vi "Host_FastOsziTest_backup.vi"() -> ()   [LabVIEW 2012]
uses:
  <vilib>/FPGAPlugInAG/PXIe-7962R/niLvFpga_Open_PXIe-7962R.vi
  <vilib>/rvi/interface/common/dynamic/niFpgaDynamicAddResources.vi
  <vilib>/Utility/error.llb/Error Cluster From Error Code.vi
  <vilib>/rvi/errors/niLvFpgaAdjustHostInterfaceError.vi
  <vilib>/FPGAPlugInAG/Dynamic/niLvFpga_Close_Dynamic.vi
  <vilib>/rvi/interface/nirviOpenFPGA/nirviOpenFPGA.xnode
  FPGA Bitfiles/AnalogIntegratorFastOszi_NI5771_PXIe-7962R.lvbitx
  <vilib>/rvi/interface/nirviReadWriteControl/nirviReadWriteControl.xnode
  <vilib>/rvi/interface/nirviMethod/nirviMethod.xnode
  <vilib>/rvi/interface/nirviCloseFPGA/nirviCloseFPGA.xnode
  <vilib>/rvi/interface/Simulation/niFpgaSimulationCallBeginRW.vi
  NiFpgaLv.dll
  <vilib>/FPGAPlugInAG/Dynamic/niLvFpga_ReadFifo_Dynamic.vi
  <vilib>/rvi/errors/niLvFpgaMergeErrorWithErrorCode.vi
  <vilib>/Analysis/NI_AALPro.lvlib
panel:
  in  "Baseline Subtract":u8=16
  in  "Pixels to Integrate":u32=10000
  in  "stop 3":bool
  out "NOT Crosstalk":dbl format="%0.2f"
  out "Crosstalk":dbl format="%0.2f"
  in  "Save?":bool
  out "time to draw(ms) 2":i32=1000
  out "Area 1":picture
  in  "stop 2":bool
  in  "sized scatter plot cosmetics 2":T1={"min size"=1, "max size"=5, "maps to max size"=5, "color array"=[16711680, 65280, 255, 16776960, 16737792, 65535]}
  in  "cartesian axis attributes 2":T2={"x minimum"=1.0, "x maximum"=500.0, "x log?"=FALSE, "x precision"=1, "x format"=enum."Decimal", "y minimum"=60.0, "y maximum"=740.0, "y log?"=FALSE, "y precision"=1, "y format"=enum."Decimal"} {"x minimum" format="%0.2f"; "x maximum" format="%0.2f"; "y minimum" format="%0.2f"; "y maximum" format="%0.2f"}
  in  "?":u16(ring)=4 items=["Points", "Squares", "Circles", "Sized Squares", "Sized-Colored Squares", "Min-Max Lines"]
  in  "line color 2":u32(colorbox)=39168
  in  "text color 2":u32(colorbox)=65280
  in  "plot color 2":u32(colorbox)=16776960
  out "time to draw(ms)":i32=1000
  out "Area 2":picture
  in  "stop":bool
  in  "sized scatter plot cosmetics":T1={"min size"=1, "max size"=5, "maps to max size"=5, "color array"=[16711680, 65280, 255, 16776960, 16737792, 65535]}
  in  "cartesian axis attributes":T2={"x minimum"=1.0, "x maximum"=500.0, "x log?"=FALSE, "x precision"=1, "x format"=enum."Decimal", "y minimum"=60.0, "y maximum"=740.0, "y log?"=FALSE, "y precision"=1, "y format"=enum."Decimal"} {"x minimum" format="%0.2f"; "x maximum" format="%0.2f"; "y minimum" format="%0.2f"; "y maximum" format="%0.2f"}
  in  "?":u16(ring)=4 items=["Points", "Squares", "Circles", "Sized Squares", "Sized-Colored Squares", "Min-Max Lines"]
  in  "line color":u32(colorbox)=39168
  in  "text color":u32(colorbox)=65280
  in  "plot color":u32(colorbox)=16776960
  out "PMT histogram":T3(graph)
  out "Mean NOT pulse length":dbl format="%0.2f"
  out "Mean pulse length":dbl format="%0.2f"
  out "NOT Laser pulse length histogram":T3(graph)
  out "Laser pulse length histogram":T3(graph)
  out "Laser (Trigger In)":i16[](graph)
  in  "Samples per Pixels":u32=10000
  out "IO Module\\AI Over Range":bool
  out "PMT (AI 0)":u8[](graph)
  # "Sampling at 1.5GHz => 0.66 ns sampling interval"
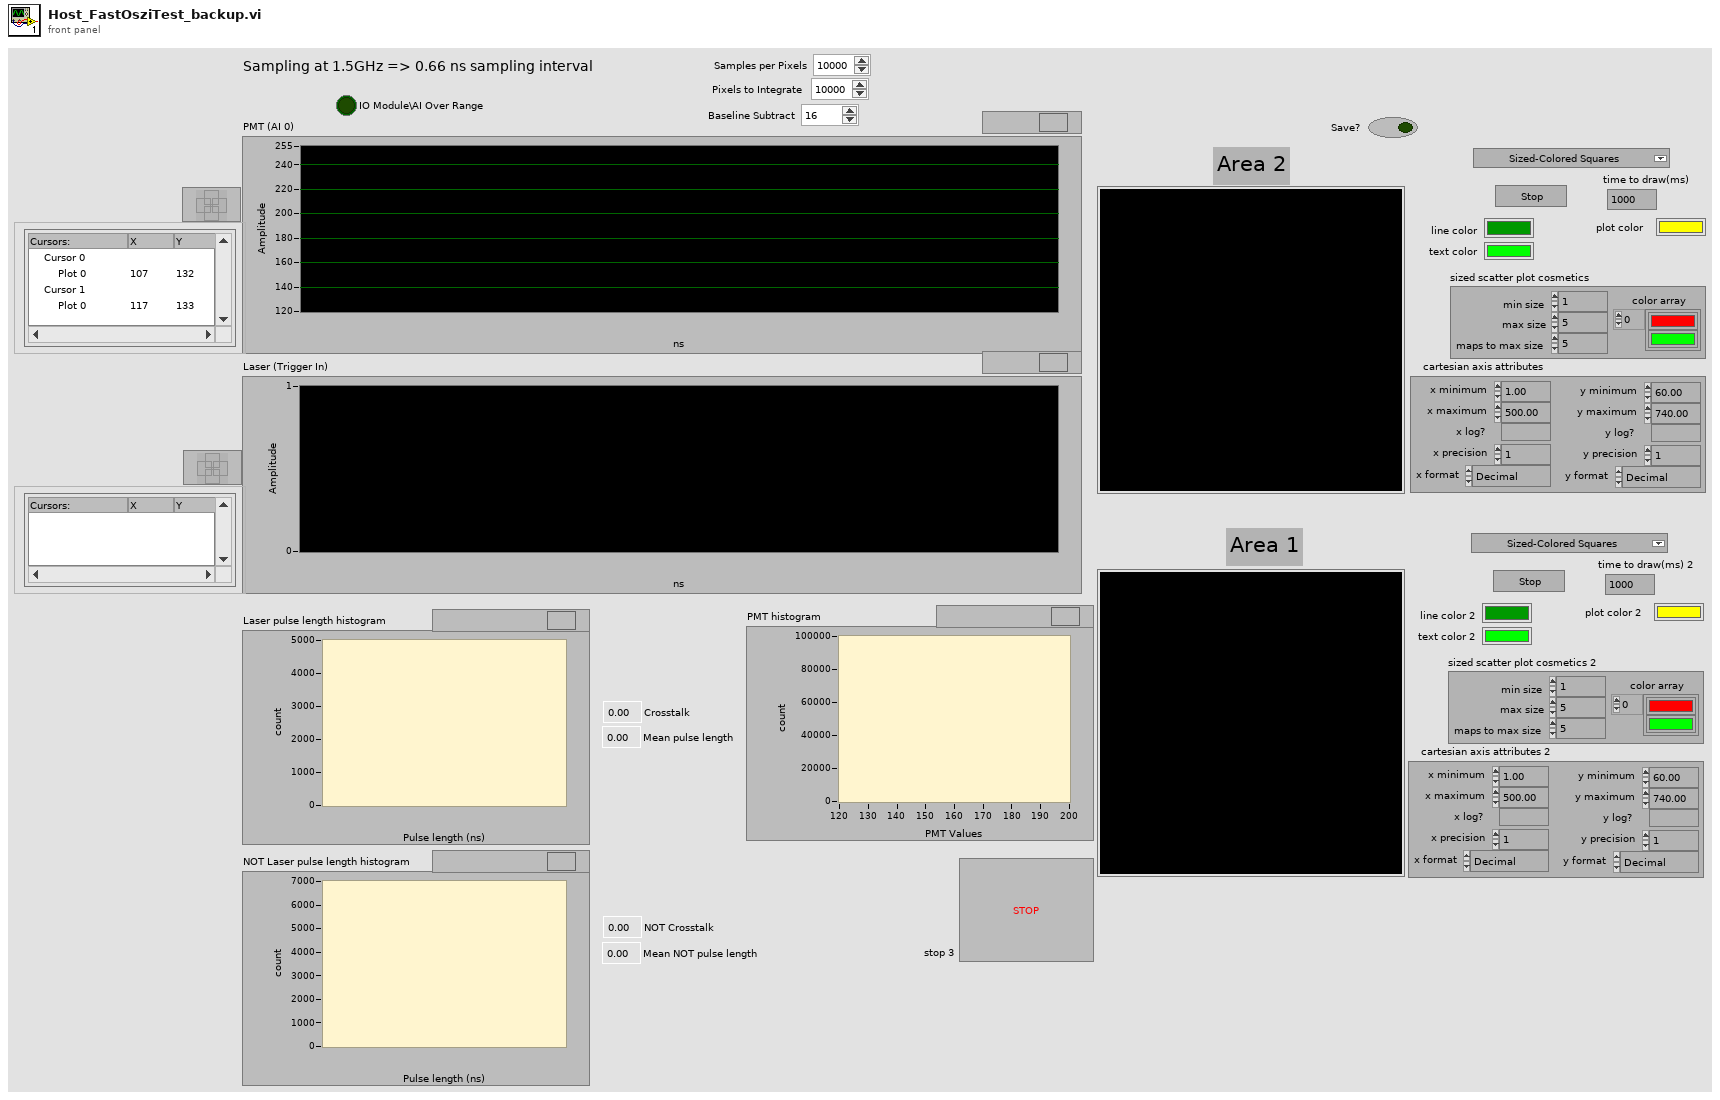
[diagram p1: front panel]
types:
  T1 = cluster{"min size":i16, "max size":i16, "maps to max size":i16, "color array":u32[]}
  T2 = cluster{"x minimum":dbl, "x maximum":dbl, "x log?":bool, "x precision":u8, "x format":enum8{"Decimal", "Scientific", "Engineering", "Binary", "Octal", "Hex"}, "y minimum":dbl, "y maximum":dbl, "y log?":bool, "y precision":u8, "y format":enum8{"Decimal", "Scientific", "Engineering", "Binary", "Octal", "Hex"}}
  T3 = cluster{"X Values":dbl[], "Histogram: h(x)":i32[]}
  T4 = cluster{"line color 2":u32, "text color 2":u32, "tick length":i16, "not crossing axes":bool, "no grids":bool}
  T5 = cluster{"plot color 2":u32, i32, "baseline(not used for these plots)":i16}
  T6 = typedef "LVBoundsTypeDef.ctl" = cluster{"Width":u32, "Height":u32}
  T7 = cluster{cluster{i32, i32, "Width":u32, "Height":u32}, "cartesian axis attributes 2":cluster{"x minimum":dbl, "x maximum":dbl, "x log?":bool, "x precision":u8, "x format":enum8{"Decimal", "Scientific", "Engineering", "Binary", "Octal", "Hex"}, "y minimum":dbl, "y maximum":dbl, "y log?":bool, "y precision":u8, "y format":enum8{"Decimal", "Scientific", "Engineering", "Binary", "Octal", "Hex"}}, cluster{"line color 2":u32, "text color 2":u32, "tick length":i16, "not crossing axes":bool, "no grids":bool}, cluster{"plot color 2":u32, i32, "baseline(not used for these plots)":i16}, "sized scatter plot cosmetics 2":cluster{"min size":i16, "max size":i16, "maps to max size":i16, "color array":u32[]}}
  T8 = cluster{"line color":u32, "text color":u32, "tick length":i16, "not crossing axes":bool, "no grids":bool}
  T9 = cluster{"plot color":u32, i32, "baseline(not used for these plots)":i16}
  T10 = cluster{cluster{i32, i32, "Width":u32, "Height":u32}, "cartesian axis attributes":cluster{"x minimum":dbl, "x maximum":dbl, "x log?":bool, "x precision":u8, "x format":enum8{"Decimal", "Scientific", "Engineering", "Binary", "Octal", "Hex"}, "y minimum":dbl, "y maximum":dbl, "y log?":bool, "y precision":u8, "y format":enum8{"Decimal", "Scientific", "Engineering", "Binary", "Octal", "Hex"}}, cluster{"line color":u32, "text color":u32, "tick length":i16, "not crossing axes":bool, "no grids":bool}, cluster{"plot color":u32, i32, "baseline(not used for these plots)":i16}, "sized scatter plot cosmetics":cluster{"min size":i16, "max size":i16, "maps to max size":i16, "color array":u32[]}}
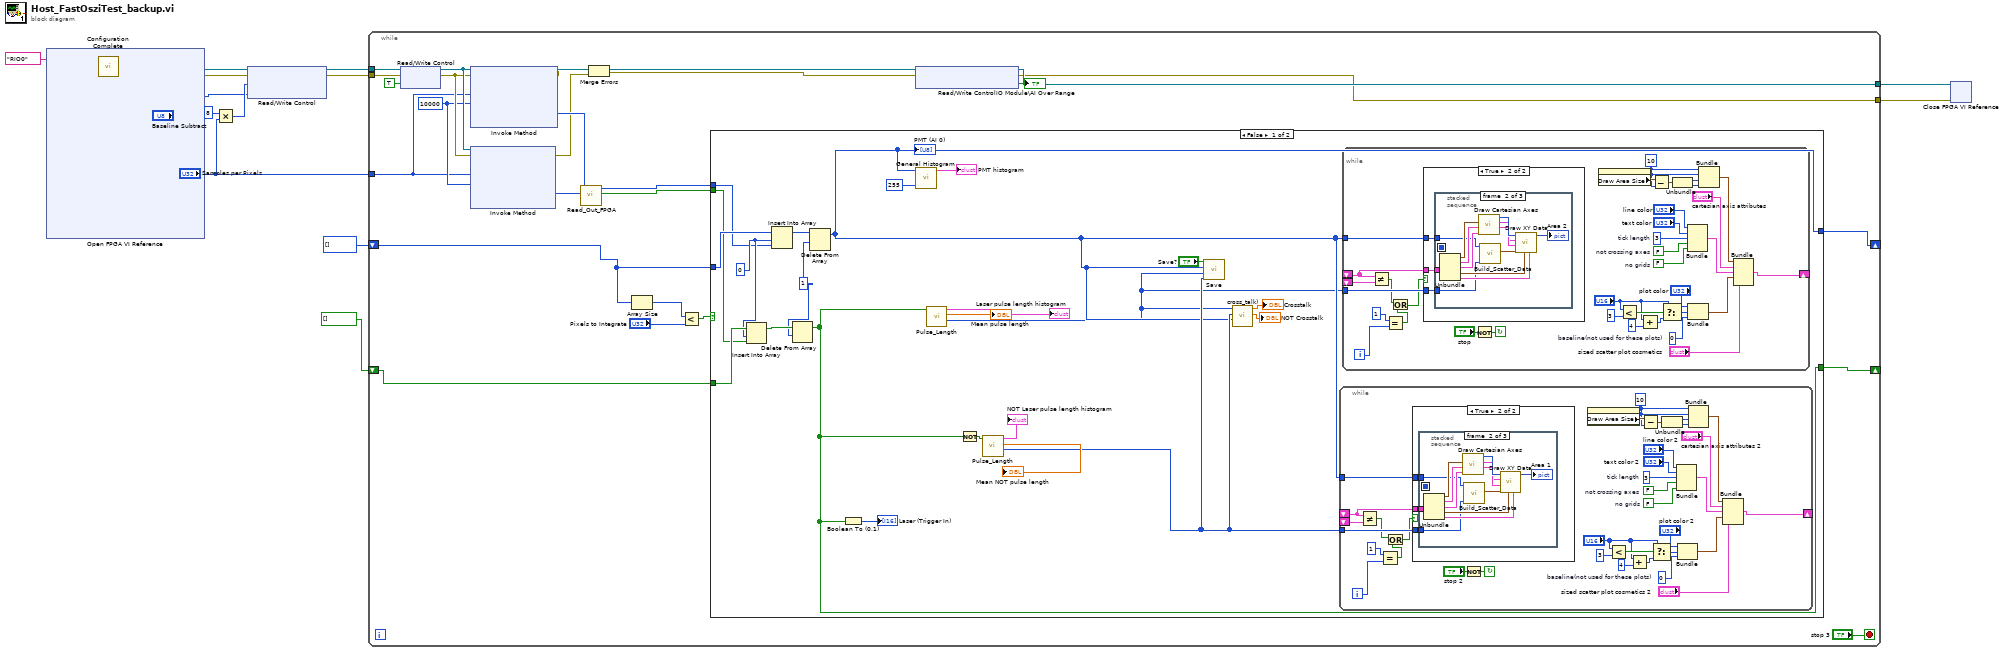
[diagram p0: block diagram]
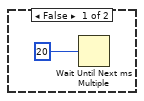
[diagram p2: hidden frame]
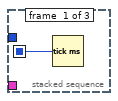
[diagram p3: hidden frame]
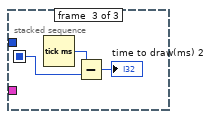
[diagram p4: hidden frame]
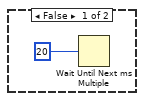
[diagram p5: hidden frame]
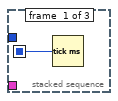
[diagram p6: hidden frame]
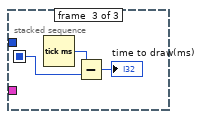
[diagram p7: hidden frame]
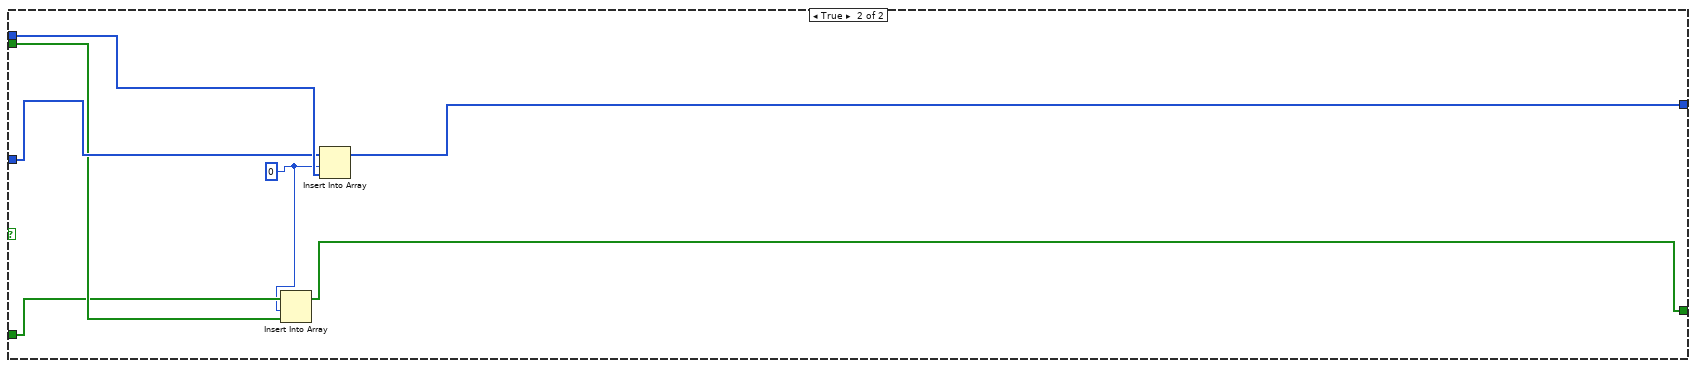
[diagram p8: hidden frame]
diagram:
  n1 = xnode "Open FPGA VI Reference"("resource name"=tag "RIO0") -> ("FPGA VI Reference Out"=w9:refnum<k20>, "error out"=w14:errorcluster)  [unwired: 1 in]
  n2 = call "Configuration Complete.vi"("error in"=w14, "FPGA VI Reference In"=w9) -> ("error out"=w12:errorcluster, "FPGA VI Reference Out"=w13:refnum<k20>)  [unwired: 7 in, 1 out]
  n3 = Multiply(x=u32 8, y="Samples per Pixels") -> (x*y=w5:u32)
  n4 = xnode "Read/Write Control"("FPGA VI Reference In"=w13, "error in"=w12, "Samples to acquire"=w5, "Baseline U8"="Baseline Subtract") -> ("FPGA VI Reference Out"=w10:refnum<k20>, "error out"=w11:errorcluster)
  n5 = while {
    tunnel: w11 -> [w41]
    tunnel: w10 -> [w40]
    tunnel: [w37] -> w8
    tunnel: [w36] -> w7
    tunnel: "Samples per Pixels" -> [w27]
    shift-right: [w17] -> _
    shift-left: u8[] [] -> [w18]
    shift-right: [w16] -> _
    shift-left: bool[] [] -> [w19]
    stop <- "stop 3" stop-if-true
    w28 = 10000 ("Timeout (ms)")
    n6 = xnode "Read/Write Control"("FPGA VI Reference In"=w40, "error in"=w41, "Acquire"=TRUE) -> ("FPGA VI Reference Out"=w33:refnum<k20>, "error out"=w32:errorcluster)
    n7 = xnode "Invoke Method"("FPGA VI Reference In"=w33, "error in"=w32, "Number of Elements"=w27, "Timeout (ms)"=w28) -> ("FPGA VI Reference Out"=w38:refnum<k20>, "error out"=w31:errorcluster, "Data"=w34:u64[])  [unwired: 1 out]
    n8 = xnode "Invoke Method"("FPGA VI Reference In"=w33, "error in"=w32, "Number of Elements"=w27, "Timeout (ms)"=w28) -> ("error out"=w29:errorcluster, "Data"=w26:u8[])  [unwired: 2 out]
    n9 = call "Read_Out_FPGA.vi"("U8ReadFIFO"=w26, "U64ReadFIFO"=w34) -> ("Trigger"=w24:bool[], "PMT Signal"=w23:u8[])  [unwired: 8 in]
    n10 = Merge Errors(w31, w29) -> (w30:errorcluster)
    n11 = Array Size(array=w18) -> (size(s)=w22:i32)
    n12 = Less?(x=w22, y="Pixels to Integrate") -> (x < y?=w20:bool)
    n13 = case shown="False" w20 {
      tunnel: w24 -> [w48 w179]
      tunnel: w23 -> [w47 w183]
      tunnel: w19 -> [w53 w178]
      tunnel: w18 -> [w54 w182]
      tunnel: [w45 w180] -> w16
      tunnel: [w46 w181] -> w17
      frame False {
        w49 = 1
        w50 = 0
        n14 = Insert Into Array(array=w53, index=w50, new element=w48) -> (w52:bool[])
        n15 = Insert Into Array(array=w54, index=w50, new element=w47) -> (w51:u8[])
        n16 = Delete From Array(array=w52, length=w49) -> (array with subset deleted=w45:bool[])  [unwired: 1 in, 1 out]
        n17 = Delete From Array(array=w51, length=w49) -> (array with subset deleted=w46:u8[])  [unwired: 1 in, 1 out]
        "PMT (AI 0)" <- w46
        n18 = Boolean To (0,1)(Boolean=w45) -> (0, 1=→"Laser (Trigger In)":i16[])
        n19 = call <vilib>:"General Histogram.vi"("X"=w46, "# bins"=255) -> ("Histogram Graph"=→"PMT histogram":T3)  [unwired: 9 in, 4 out]
        n20 = call "Pulse_Length.vi"("Trigger"=w45) -> ("Rising Index"=w42:i32[], "Mean Pulse Length"=→"Mean pulse length":dbl, "Histogram Graph"=→"Laser pulse length histogram":T3)  [unwired: 8 in]
        n21 = Not(x=w45) -> (.not. x?=w63:bool[])
        n22 = call "Pulse_Length.vi"("Trigger"=w63) -> ("Rising Index"=w55:i32[], "Mean Pulse Length"=→"Mean NOT pulse length":dbl, "Histogram Graph"=→"NOT Laser pulse length histogram":T3)  [unwired: 8 in]
        n23 = call "Save.vi"("Rising Index 1"=w55, "Rising Index 2"=w42, "PMT (AI 0)"=w46, "Save?"="Save?") -> ()  [unwired: 8 in]
        n24 = call "cross_talk).vi"("Array"=w46, "Rising Index 2"=w55, "Rising Index"=w42) -> ("x/y 2"=→"NOT Crosstalk":dbl, "x/y"=→"Crosstalk":dbl)  [unwired: 7 in]
        n25 = while {
          shift-left: _ -> [w73]
          shift-left: _ -> [w72]
          shift-right: [w74] -> _
          tunnel: w46 -> [w71]
          tunnel: w55 -> [w70]
          i -> [w68]
          stop <- w98 continue-if-true
          w82 = i16 0  # baseline(not used for these plots)
          w89 = FALSE  # not crossing axes
          w90 = i16 3  # tick length
          w88 = FALSE  # no grids
          w93 = 10
          n26 = Not Equal?(x=w72, y=w73) -> (x != y?=w67:bool)
          n27 = Equal?(x=1, y=w68) -> (x = y?=w66:bool)
          n28 = Or(x=w67, y=w66) -> (x .or. y?=w65:bool)
          n29 = case shown="True" w65 {
            tunnel: w72 -> [_ w103]
            tunnel: w71 -> [_ w102]
            tunnel: w70 -> [_ w101]
            frame False {
              n30 = Wait Until Next ms Multiple(millisecond multiple=20) -> ()  [unwired: 1 out]
            }
            frame True {
              n31 = stacked-sequence {
                seq-local: [w104 _ _] -> [_ _ w119]
                tunnel: w103 -> [_ w111 _]
                tunnel: w102 -> [_ w106 _]
                tunnel: w101 -> [_ w105 _]
                frame #0 {
                  n32 = Tick Count (ms)() -> (millisecond timer value=w104:u32)
                }
                frame #1 {
                  n33 = Unbundle(w111) -> (w112:cluster{i32, i32, "Width":u32, "Height":u32}, "cartesian axis attributes 2"=w113:T2, w114:T4, w109:T5, "sized scatter plot cosmetics 2"=w108:T1)
                  n34 = call <vilib>:"Draw Cartesian Axes.vi"("grid cosmetics"=w114, "axis attributes"=w113, "bounding rect"=w112) -> ("y scale factors"=w116:cluster{"a":dbl, "b":dbl, "log?":bool}, "x scale factors"=w115:cluster{"a":dbl, "b":dbl, "log?":bool}, "new picture"=w117:picture)  [unwired: 6 in]
                  n35 = call "Build_Scatter_Data.vi"("Rising Index"=w105, "PMT (AI 0)"=w106) -> ("data"=w107:cluster{"x":dbl, "y":dbl}[])  [unwired: 9 in]
                  n36 = call <vilib>:"Draw XY Data.vi"("[sized scatter plot cosmetics]"=w108, "xy cosmetics"=w109, "xy data"=w107, "y scale factors"=w116, "x scale factors"=w115, "picture"=w117) -> ("new picture"=→"Area 1":picture)  [unwired: 5 in]
                }
                frame #2 {
                  n37 = Tick Count (ms)() -> (millisecond timer value=w120:u32)
                  n38 = Subtract(x=w120, y=w119) -> (x-y=→"time to draw(ms) 2":u32)
                }
              }
            }
          }
          n39 = Not(x="stop 2") -> (.not. x?=w98:bool)
          n40 = property on="Area 1" class="Pict"() -> ("Draw Area Size"=w97:T6)  [unwired: 2 in, 2 out]
          n41 = Less?(x="?", y=3) -> (x < y?=w87:bool)
          n42 = Add(x="?", y=4) -> (x+y=w85:i32)
          n43 = Subtract(x=w97, y=w93) -> (x-y=w96:T6)
          n44 = Select(t="?", s=w87, f=w85) -> (s? t:f=w83:i32)
          n45 = Unbundle(w96) -> ("Width"=w94:u32, "Height"=w95:u32)
          n46 = Bundle("line color 2"="line color 2", "text color 2"="text color 2", "tick length"=w90, "not crossing axes"=w89, "no grids"=w88) -> (w77:T4)  [unwired: 1 in]
          n47 = Bundle("plot color 2"="plot color 2", w83, "baseline(not used for these plots)"=w82) -> (w78:T5)  [unwired: 1 in]
          n48 = Bundle(w93, w93, "Width"=w94, "Height"=w95) -> (w75:cluster{i32, i32, "Width":u32, "Height":u32})  [unwired: 1 in]
          n49 = Bundle(w75, "cartesian axis attributes 2"="cartesian axis attributes 2", w77, w78, "sized scatter plot cosmetics 2"="sized scatter plot cosmetics 2") -> (w74:T7)  [unwired: 1 in]
        }
        n50 = while {
          shift-left: _ -> [w129]
          shift-left: _ -> [w128]
          shift-right: [w130] -> _
          tunnel: w46 -> [w127]
          tunnel: w42 -> [w126]
          i -> [w123]
          stop <- w154 continue-if-true
          w138 = i16 0  # baseline(not used for these plots)
          w145 = FALSE  # not crossing axes
          w146 = i16 3  # tick length
          w144 = FALSE  # no grids
          w149 = 10
          n51 = Not Equal?(x=w128, y=w129) -> (x != y?=w122:bool)
          n52 = Equal?(x=1, y=w123) -> (x = y?=w124:bool)
          n53 = Or(x=w122, y=w124) -> (x .or. y?=w121:bool)
          n54 = case shown="True" w121 {
            tunnel: w128 -> [_ w159]
            tunnel: w127 -> [_ w158]
            tunnel: w126 -> [_ w157]
            frame False {
              n55 = Wait Until Next ms Multiple(millisecond multiple=20) -> ()  [unwired: 1 out]
            }
            frame True {
              n56 = stacked-sequence {
                seq-local: [w160 _ _] -> [_ _ w175]
                tunnel: w159 -> [_ w167 _]
                tunnel: w158 -> [_ w162 _]
                tunnel: w157 -> [_ w161 _]
                frame #0 {
                  n57 = Tick Count (ms)() -> (millisecond timer value=w160:u32)
                }
                frame #1 {
                  n58 = Unbundle(w167) -> (w168:cluster{i32, i32, "Width":u32, "Height":u32}, "cartesian axis attributes"=w169:T2, w170:T8, w165:T9, "sized scatter plot cosmetics"=w164:T1)
                  n59 = call <vilib>:"Draw Cartesian Axes.vi"("grid cosmetics"=w170, "axis attributes"=w169, "bounding rect"=w168) -> ("y scale factors"=w172:cluster{"a":dbl, "b":dbl, "log?":bool}, "x scale factors"=w171:cluster{"a":dbl, "b":dbl, "log?":bool}, "new picture"=w173:picture)  [unwired: 6 in]
                  n60 = call "Build_Scatter_Data.vi"("Rising Index"=w161, "PMT (AI 0)"=w162) -> ("data"=w163:cluster{"x":dbl, "y":dbl}[])  [unwired: 9 in]
                  n61 = call <vilib>:"Draw XY Data.vi"("[sized scatter plot cosmetics]"=w164, "xy cosmetics"=w165, "xy data"=w163, "y scale factors"=w172, "x scale factors"=w171, "picture"=w173) -> ("new picture"=→"Area 2":picture)  [unwired: 5 in]
                }
                frame #2 {
                  n62 = Tick Count (ms)() -> (millisecond timer value=w176:u32)
                  n63 = Subtract(x=w176, y=w175) -> (x-y=→"time to draw(ms)":u32)
                }
              }
            }
          }
          n64 = Not(x="stop") -> (.not. x?=w154:bool)
          n65 = property on="Area 2" class="Pict"() -> ("Draw Area Size"=w153:T6)  [unwired: 2 in, 2 out]
          n66 = Less?(x="?", y=3) -> (x < y?=w143:bool)
          n67 = Add(x="?", y=4) -> (x+y=w141:i32)
          n68 = Subtract(x=w153, y=w149) -> (x-y=w152:T6)
          n69 = Select(t="?", s=w143, f=w141) -> (s? t:f=w139:i32)
          n70 = Unbundle(w152) -> ("Width"=w150:u32, "Height"=w151:u32)
          n71 = Bundle("line color"="line color", "text color"="text color", "tick length"=w146, "not crossing axes"=w145, "no grids"=w144) -> (w133:T8)  [unwired: 1 in]
          n72 = Bundle("plot color"="plot color", w139, "baseline(not used for these plots)"=w138) -> (w134:T9)  [unwired: 1 in]
          n73 = Bundle(w149, w149, "Width"=w150, "Height"=w151) -> (w131:cluster{i32, i32, "Width":u32, "Height":u32})  [unwired: 1 in]
          n74 = Bundle(w131, "cartesian axis attributes"="cartesian axis attributes", w133, w134, "sized scatter plot cosmetics"="sized scatter plot cosmetics") -> (w130:T10)  [unwired: 1 in]
        }
      }
      frame True {
        w177 = 0
        n75 = Insert Into Array(array=w178, index=w177, new element=w179) -> (w180:bool[])
        n76 = Insert Into Array(array=w182, index=w177, new element=w183) -> (w181:u8[])
      }
    }
    n77 = xnode "Read/Write Control"("FPGA VI Reference In"=w38, "error in"=w30) -> ("FPGA VI Reference Out"=w37:refnum<k20>, "error out"=w36:errorcluster, "IO Module\\AI Over Range"=→"IO Module\\AI Over Range":bool)
  }
  n78 = xnode "Close FPGA VI Reference"("FPGA VI Reference In"=w8, "error in"=w7) -> ()  [unwired: 1 out]
